vi "Run Test Case and Get Case Result.vi"(8 "error in (no error)":errorcluster, 11 "Error First Test Case in":refnum<class "LUnit Test Case.lvclass">) -> (0 "error out":errorcluster, 3 "Test Case Result out":T1)   [LabVIEW 2020, in "LUnit Tests.lvlib" / "Test Case Result Test.lvclass"]
uses:
  Test Case Result Test.lvclass
  source/Framework/Test Case/LUnit Test Case.lvclass
  source/Framework/Result Types/Case Result/Test Case Result.ctl
  source/Framework/Result Types/Method Result/Method Result.ctl
  source/Framework/Result Types/Assertion Result/Public/TypeDefs/Status.ctl
  source/Framework/Result Types/Assertion Result/Assertion Result.ctl
  source/Framework/Result Types/Assertion Result/Public/TypeDefs/Assertion Type.ctl
  source/Framework/Execution API/Execution API.lvclass
  source/Framework/Result Types/Assertion Result/Assertion Result.lvlib
  source/Framework/Result Types/Method Result/Method Result.lvlib
  source/Framework/Result Types/Case Result/Test Case Result.lvlib
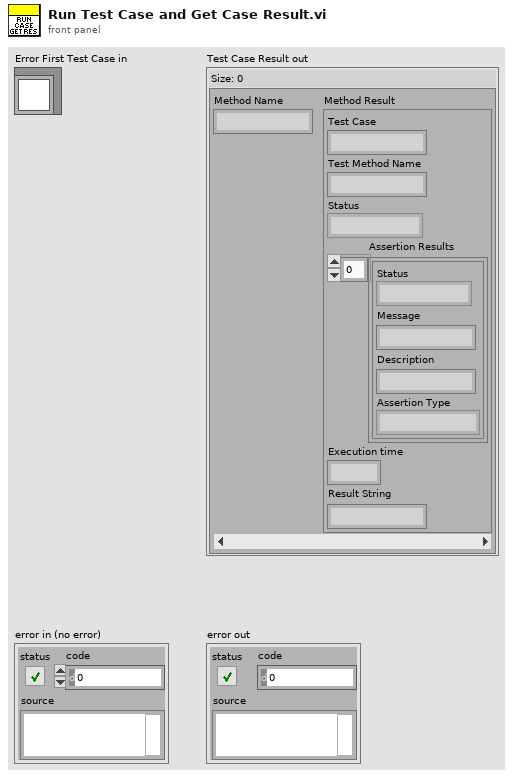
[diagram p1: front panel]
types:
  T1 = typedef "Test Case Result.lvlib/Test Case Result.ctl" = map{string, T2}
  T2 = typedef "Method Result.lvlib/Method Result.ctl" = cluster{"Test Case":string, "Test Method Name":string, "Status":T3, "Assertion Results":T4[], "Execution time":dbl, "Result String":string}
  T3 = typedef "Assertion Result.lvlib/Status.ctl" = enum16{"Pass", "Fail", "Error", "Skipped", "Setup Error", "Broken", "Teardown Error"}
  T4 = typedef "Assertion Result.lvlib/Assertion Result.ctl" = cluster{"Status":T3, "Message":string, "Description":string, "Assertion Type":T5}
  T5 = typedef "Assertion Result.lvlib/Assertion Type.ctl" = enum16{"None", "Pass", "Fail", "Skip", "Pass if Equal", "Fail if Equal", "Pass if Error", "Fail if Error", "Pass if", "Fail if"}
  T6 = cluster{"Result Events":refnum<event-registration>, "Event Registration Refnum":refnum<event-registration>}
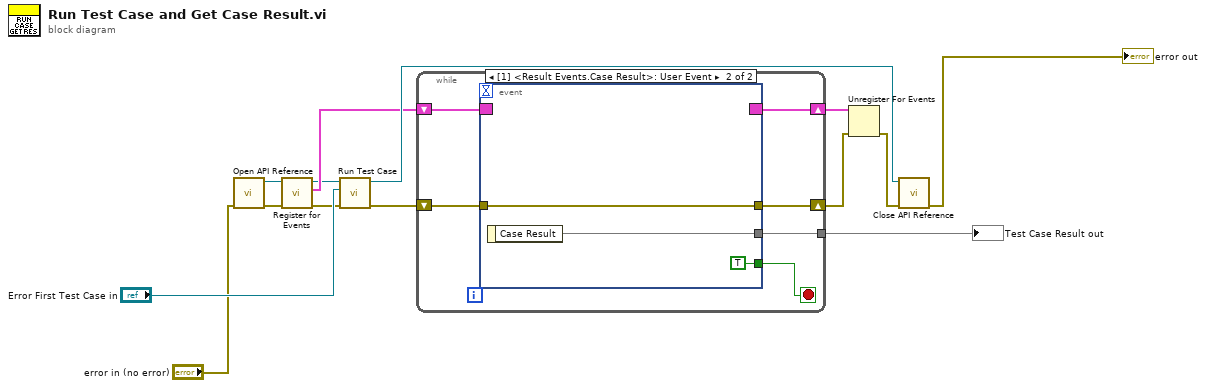
[diagram p0: block diagram]
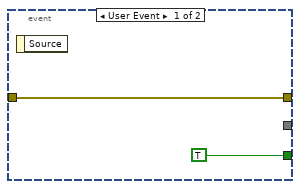
[diagram p2: hidden frame]
diagram:
  n1 = call "Open API Reference.vi"("error in (no error)"="error in (no error)") -> ("error out"=w3:errorcluster, "Execution API out"=w2:refnum<class "Execution API.lvclass">)  [unwired: 9 in]
  n2 = call "Register for Events.vi"("error in (no error)"=w3, "Execution API In"=w2) -> ("error out"=w5:errorcluster, "Result Registration Refnum"=w6:T6, "Execution API Out"=w4:refnum<class "Execution API.lvclass">)  [unwired: 7 in]
  n3 = call "Run Test Case.vi"("error in (no error)"=w5, "Test Case"="Error First Test Case in", "Execution API In"=w4) -> ("error out"=w8:errorcluster, "Execution API Out"=w11:refnum<class "Execution API.lvclass">)  [unwired: 7 in]
  n4 = while {
    shift-right: [w19] -> w7
    shift-left: w6 -> [w20]
    shift-right: [w17] -> w9
    shift-left: w8 -> [w18]
    tunnel: [w15] -> w1
    stop <- w16 stop-if-true
    n5 = event shown="[1] <Result Events.Case Result>: User Event" {
      selector: w20 -> [_ _]
      dyn-events: [_ _] -> w19
      timeout: _ -> [_ _]
      tunnel: w18 -> [w22 w25]
      tunnel: [w22 w25] -> w17
      tunnel: [TRUE TRUE] -> w16
      tunnel: [_ w23] -> w15
      event User Event {
        n6 = event-data() -> ()  [unwired: 1 in, 1 out]
      }
      event User Event {
        n7 = event-data() -> ("Case Result"=w23:T1)  [unwired: 1 in]
      }
    }
  }
  "Test Case Result out" <- w1
  n8 = Unregister For Events(event registration refnum=w7, error in=w9) -> (error out=w10:errorcluster)
  n9 = call "Close API Reference.vi"("error in (no error)"=w10, "Execution API in"=w11) -> ("error out"=→"error out":errorcluster)  [unwired: 9 in]
